vi "picoquant_close_dset.vi"(8 "error in (no error)":errorcluster, 11 "hydraharp in":refnum<class "hydraharp.lvclass">) -> (0 "error out":errorcluster, 3 "hydraharp out":refnum<class "hydraharp.lvclass">)   [LabVIEW 2015, in "hydraharp.lvclass"]
uses:
  hydraharp.lvclass
  hydraharp.lvclass/hydraharp.ctl
  Data Logger Class/data_logger.lvclass
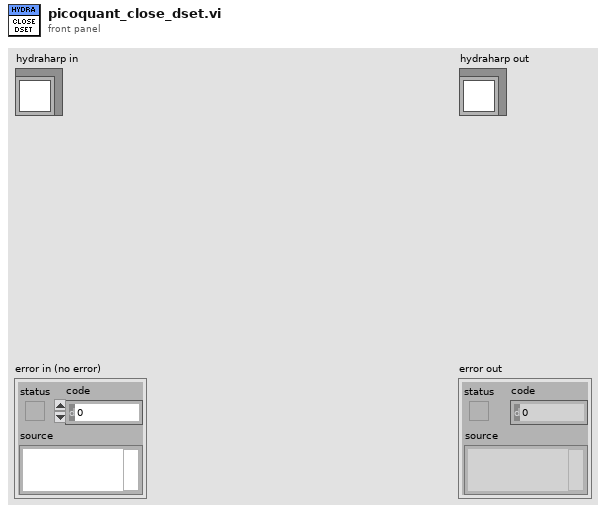
[diagram p1: front panel]
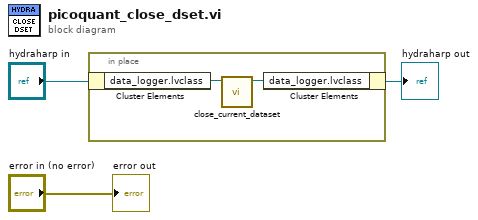
[diagram p0: block diagram]
diagram:
  n1 = in-place {
    n2 = in-place-cluster #1("hydraharp in") -> ("data_logger.lvclass"=w5:refnum<class "data_logger.lvclass">)
    n3 = call-dynamic "close_current_dataset.vi"("data_logger in"=w5) -> ("data_logger out"=w4:refnum<class "data_logger.lvclass">)  [unwired: 9 in, 1 out]
    n4 = in-place-cluster #1("data_logger.lvclass"=w4) -> (→"hydraharp out":refnum<class "hydraharp.lvclass">)
  }
  "error out" <- "error in (no error)"
